vi "Configure Serial Output Power Over Coax Sink.vi"(0 "fpga interface in":refnum<k20>, 5 "serial output channels":string[](array[string]), 7 "power over coax sink":i32(ring) items=["None"=0, "Auxiliary"=2], 9 "power over coax in range timeout (s)":dbl=5.0, 11 "error in (no error)":errorcluster) -> (4 "fpga interface out":refnum<k20>, 6 "power over coax sink in range":bool[](array[boolean]), 15 "error out":errorcluster)   [LabVIEW 2023, in "GettingStarted_Common_148X_Host.lvlib"]
uses:
  GettingStarted_Common_148X_Host.lvlib
  <instrlib>/FlexRIO/API/Host/v1/NI FlexRIO/API/Get Property Reference - Fpga Small.vi
  <resource>/objmgr/niflexrioapiChannel.rc
  <instrlib>/FlexRIO/API/Host/v1/NI FlexRIO API v1.lvlib
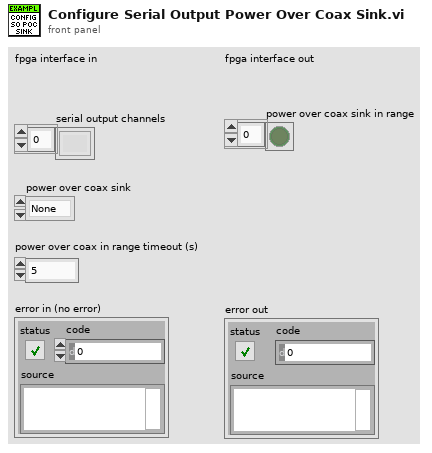
[diagram p1: front panel]
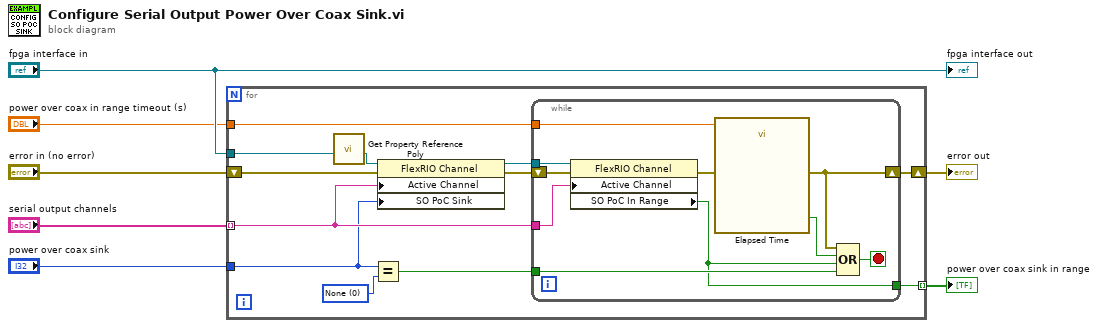
[diagram p0: block diagram]
diagram:
  n1 = for {
    tunnel: "fpga interface in" -> [w19]
    tunnel: "serial output channels" -> [w17] mode=indexing
    shift-right: [w14] -> w5
    shift-left: "error in (no error)" -> [w18]
    tunnel: "power over coax sink" -> [w8]
    tunnel: "power over coax in range timeout (s)" -> [w10]
    tunnel: [w9] -> w1 mode=indexing
    w12 = 0 items=["None", "Internal", "Auxiliary"] ("Serial Input Power Over Coax Source 2")
    n2 = call-poly <instrlib>:"Get Property Reference Poly.vi"("fpga interface in"=w19) -> ("property reference"=w11:refnum<k20>)  [unwired: 5 in, 2 out]
    n3 = Equal?(x=w8, y=w12) -> (x = y?=w13:bool)
    n4 = property class="FlexRIO Channel"(reference=w11, error in=w18, "Active Channel"=w17, "SO PoC Sink"=w8) -> (reference out=w16:refnum<k20>, error out=w15:errorcluster)
    n5 = while {
      tunnel: w16 -> [w28]
      tunnel: w17 -> [w27]
      tunnel: w13 -> [w25]
      shift-right: [w20] -> w14
      shift-left: w15 -> [w29]
      tunnel: w10 -> [w22]
      tunnel: [w21] -> w9
      stop <- w26 stop-if-true
      n6 = property class="FlexRIO Channel"(reference=w28, error in=w29, "Active Channel"=w27) -> (error out=w24:errorcluster, "SO PoC In Range"=w21:bool)  [unwired: 1 out]
      n7 = call "Elapsed Time"("Time Target (s)"=w22, "error in (no error)"=w24) -> ("Time has Elapsed"=w23:bool, "error out"=w20:errorcluster)  [unwired: 10 in, 6 out]
      n8 = Compound Arithmetic op=OR(w20, w23, w21, w25) -> (w26:bool)
    }
  }
  "error out" <- w5
  "power over coax sink in range" <- w1
  "fpga interface out" <- "fpga interface in"
